vi "Teleop.vi"(10 "Match Info":T1={"Autonomous Elapsed Seconds"=0.0, "TeleOp Elapsed Seconds"=0.0, "Disabled Elapsed Seconds"=0.0, "Visited Autonomous"=FALSE, "Visited TeleOp"=FALSE, "Visited Disabled"=FALSE, "Autonomous Settings"={"Autonomous Style"=enum."Independent", "VI Refnum"=refnum}}, 11 "Call Context":T2) -> ()   [LabVIEW 2016]
doc: "This VI is called for each TeleOp packet received from the DS where the robot is not disabled. It is often used to read from the joysticks and update I/O or to update setpoints for timed control loops. It should complete and return within 20 milliseconds or it may miss DS packets."
uses:
  <vilib>/Rock Robotics/WPI/DriverStation/WPI_DriverStationDerivedRobotMode.ctl
  <vilib>/Rock Robotics/WPI/DriverStation/WPI_DriverStationMatch Info.ctl
  <vilib>/Rock Robotics/WPI/ThirdParty/CanMotor/TalonSRX/WPI_CANTalonSRX_APIFeedbackSelect.ctl
  <vilib>/Rock Robotics/WPI/ThirdParty/CanMotor/TalonSRX/WPI_CANTalonSRX_APIControlMode.ctl
  <vilib>/Rock Robotics/WPI/Utilities/WPI_GetSetVariantRefNum.vi
panel:
  out "SensorPosRotations":dbl
  out "Motor output Plot":cluster{"Applied Throttle":dbl}(graph)
  out "Target RPM":dbl
  out "SensorRPM Velocity RPM":dbl
  in  "Ramp Rate":dbl
  in  "I Zone":dbl
  in  "F":dbl
  in  "D":dbl
  in  "I":dbl
  in  "P":dbl
  out "Applied Output":dbl
  out "Speed Closed Loop Plots":cluster{dbl, "Sensor Velocity":dbl}(graph)
  # "Use the Left Y-axis on Logitech Gamepad.\n\nVelocityNativeUnits = Change In Sensor / 100mS\nalso\nVelocityNativeUnits = RPM / 600 * SensorUnitsPerRotation\n\nFgain = 100% X 1023 / VelocityNativeUnits , \n       where VelocityNativeUnits  is measured at 100% throttle\n\nMag Encoder has 4096 units per rotation.\n\nExample: VelocityRPM is 10198 at 100% throttle\n                 => VelocityNativeUnits = (10198 / 600 * 4096) = 69618\n                 => Fgain = (1023 / 69618)  = 0.01469"
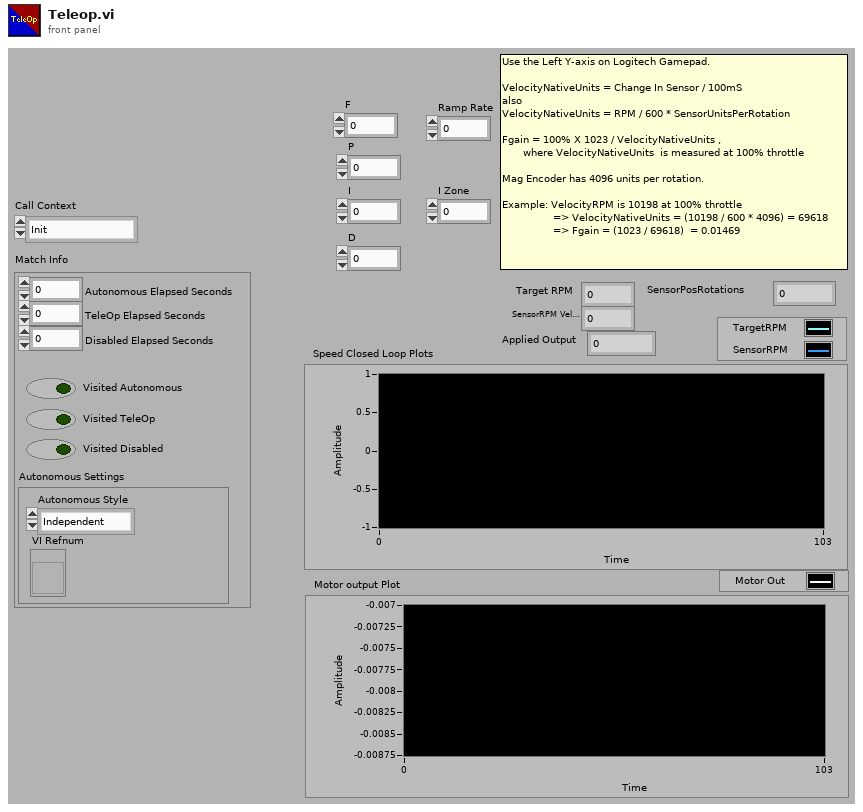
[diagram p1: front panel]
types:
  T1 = typedef "WPI_DriverStationMatch Info.ctl" = cluster{"Autonomous Elapsed Seconds":dbl, "TeleOp Elapsed Seconds":dbl, "Disabled Elapsed Seconds":dbl, "Visited Autonomous":bool, "Visited TeleOp":bool, "Visited Disabled":bool, "Autonomous Settings":cluster{"Autonomous Style":enum16{"Iterative", "Independent"}, "VI Refnum":refnum<vi>}}
  T2 = typedef "WPI_DriverStationDerivedRobotMode.ctl" = enum16{"Init", "Execute", "Stop"}
  T3 = typedef "WPI_CANTalonSRX_APIFeedbackSelect.ctl" = enum16{"Digital Quadrature Encoder", "Analog Potentiometer", "Analog Encoder", "Count on Quad-A (Rising-Edge)", "Count on Quad-A (Falling-Edge)", "CTR Magnetic Enc (Absolute)", "CTR Magnetic Enc (Relative)", "Pulse Width"}
  T4 = typedef "WPI_MotorControlDeviceRef.ctl" = cluster{"DeviceStatus":errorcluster, "Type":T5, "PWM":cluster{"PWM Channel":T6, "DeadBand":T7}, "CAN":cluster{"Device Number":u8, "SetOutput VI Ref":variant, "GetOutput VI Ref":variant, "Enable VI Ref":variant, "Disable VI Ref":variant, "Data":variant}, "Invert":bool}
  T5 = typedef "WPI_MotorControlType.ctl" = enum16{"PWM", "CAN"}
  T6 = typedef "FPGA_DIOPWMChannel.ctl" = enum8{"PWM 0", "PWM 1", "PWM 2", "PWM 3", "PWM 4", "PWM 5", "PWM 6", "PWM 7", "PWM 8", "PWM 9", "PWM MXP 0", "PWM MXP 1", "PWM MXP 2", "PWM MXP 3", "PWM MXP 4", "PWM MXP 5", "PWM MXP 6", "PWM MXP 7", "PWM MXP 8", "PWM MXP 9", "Invalid"}
  T7 = typedef "WPI_PWMDeadband.ctl" = cluster{"Name":string, "maxPositivePwm":i32, "minPositivePwm":i32, "centerPwm":i32, "maxNegativePwm":i32, "minNegativePwm":i32, "angularRange":u16}
  T8 = typedef "WPI_JoystickDevRef.ctl" = cluster{"Device":T9}
  T9 = typedef "WPI_JoystickDeviceEnum.ctl" = enum16{"USB 0", "USB 1", "USB 2", "USB 3", "USB 4", "USB 5"}
  T10 = typedef "WPI_CANTalonSRX_APIControlMode.ctl" = enum8{"Percent VBus", "Speed", "Position", "Slave", "Unchanged / Invalid", "Voltage Compensation", "Current", "Motion Profile", "Motion Magic"}
  T11 = typedef "WPI_CANTalonSRX_GlobalStatus.ctl" = cluster{"Applied Throttle":dbl, "Module Enabled":bool, "CAN Error":errorcluster, "Closed Loop Error":dbl, "Forward Limit Switch Closed":bool, "Reverse Limit Switch Closed":bool, "Sensor Position":dbl, "Sensor Velocity":dbl, "Current":dbl, "Sticky Fault - Over Temp":bool, "Sticky Fault - Under Voltage":bool, "Sticky Fault - Forward Limit":bool, "Sticky Fault - Reverse Limit":bool, "Sticky Fault - Forward Soft Limit":bool, "Sticky Fault - Reverse Soft Limit":bool, "Brake is Enabled":bool, "Encoder Position":dbl, "Encoder Velocity":dbl, "Encoder Index Count":dbl, "Encoder A Pin State":bool, "Encoder B Pin State":bool, "Encoder Index Pin State":bool, "Analog In":dbl, "Analog In Velocity":dbl, "Temperature (C)":dbl, "Battery Voltage":dbl, "Control 5 Is Supported":bool, "Current Profile Slot Select":dbl, "Pos Div 8":bool, "Vel Div 4":bool, "Pulse Width Position":i32, "Pulse Width Velocity":i32, "Pulse Width Rise To Rise (us)":i32, "Pulse Width Rise To Fall (us)":i32, "Mot Prof Active Is Under Run":bool, "Mot Prof Active Has Under Run":bool, "Mot Prof Active Is Last":bool, "Mot Prof Active Velocity Only":bool, "Mot Prof Active Is Valid":bool, "Mot Prof Buffer Is Full":bool, "Mot Prof Active Profile Slot Select":i32, "Mot Prof NextID":i32, "Mot Prof Count":i32, "Mot Prof Active Velocity":dbl, "Mot Prof Active Position":dbl, "Mot Prof Output Enable":i32, "UsageFrame":u32}
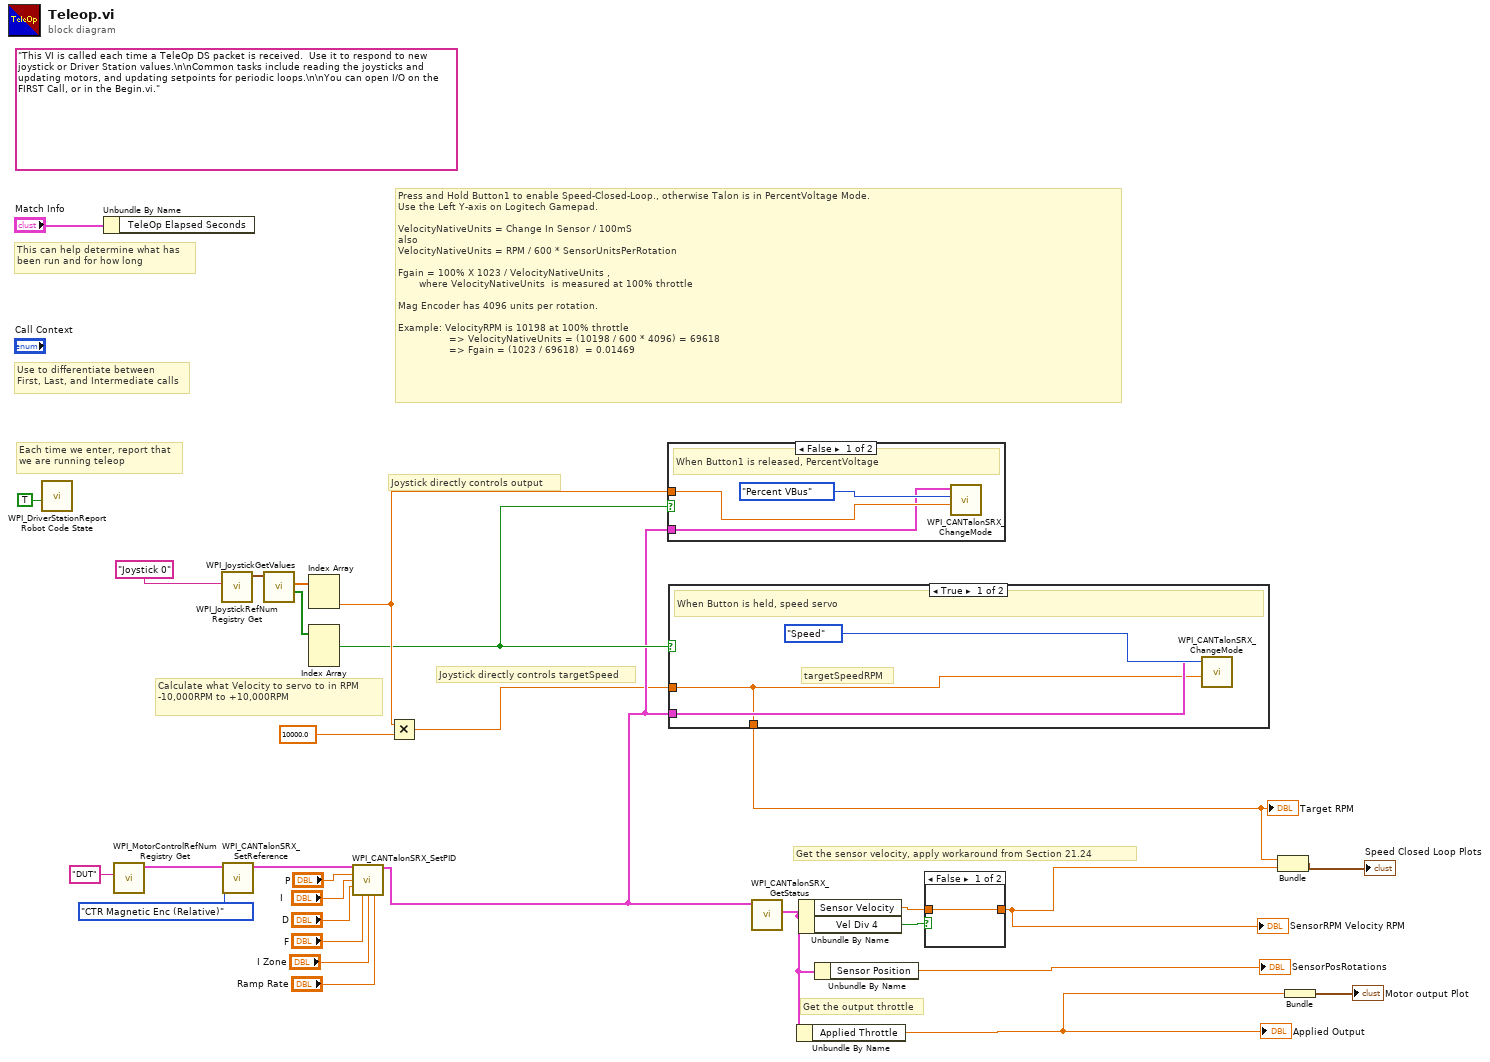
[diagram p0: block diagram]
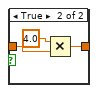
[diagram p2: hidden frame]
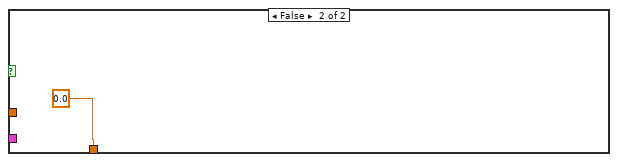
[diagram p4: hidden frame]
diagram:
  (unwired) "This VI is called each time a TeleOp DS packet is received.  Use it to respond to new joystick or Driver Station values.\n\nCommon tasks include reading the joysticks and updating motors, and updating setpoints for periodic loops.\n\nYou can open I/O on the FIRST Call, or in the Begin.vi."
  # "Press and Hold Button1 to enable Speed-Closed-Loop., otherwise Talon is in PercentVoltage Mode.  \nUse the Left Y-axis on Logitech Gamepad.\n\nVelocityNativeUnits = Change In Sensor / 100mS\nalso\nVelocityNativeUnits = RPM / 600 * SensorUnitsPerRotation\n\nFgain = 100% X 1023 / VelocityNativeUnits , \n       where VelocityNativeUnits  is measured at 100% throttle\n\nMag Encoder has 4096 units per rotation.\n\nExample: VelocityRPM is 10198 at 100% throttle\n                 => VelocityNativeUnits = (10198 / 600 * 4096) = 69618\n                 => Fgain = (1023 / 69618)  = 0.01469"
  # "Get the output throttle"
  # "Get the sensor velocity, apply workaround from Section 21.24"
  # "Joystick directly controls targetSpeed"
  # "Joystick directly controls output"
  # "Calculate what Velocity to servo to in RPM\n-10,000RPM to +10,000RPM"
  # "Each time we enter, report that\nwe are running teleop"
  # "Use to differentiate between\nFirst, Last, and Intermediate calls"
  # "This can help determine what has\nbeen run and for how long"
  n1 = call <vilib>:"WPI_DriverStationReport Robot Code State.vi"("TeleOp"=TRUE ("Autonomous")) -> ()  [unwired: 10 in, 1 out]
  n2 = Unbundle By Name("Match Info") -> ()  [unwired: 1 out]
  n3 = call <vilib>:"WPI_MotorControlRefNum Registry Get.vi"("refnum name"="DUT") -> ("MotorControlDevRef"=w10:T4)  [unwired: 9 in, 1 out]
  n4 = call <vilib>:"WPI_JoystickRefNum Registry Get.vi"("refnum name"="Joystick 0") -> ("JoystickDevRef"=w28:T8)  [unwired: 1 in, 9 out]
  n5 = call <vilib>:"WPI_CANTalonSRX_SetReference.vi"("Feedback Reference"=WPI_CANTalonSRX_APIFeedbackSelect."CTR Magnetic Enc (Relative)", "CAN Talon SRX Ref"=w10) -> ("CAN Talon SRX Ref"=w9:T4)  [unwired: 8 in, 1 out]
  n6 = call <vilib>:"WPI_JoystickGetValues.vi"("JoystickDevRef"=w28) -> ("Buttons"=w25:bool[], "Axes"=w26:dbl[])  [unwired: 6 in, 3 out]
  n7 = Index Array(array=w26) -> (element #2=w17:dbl)  [unwired: 2 in, 1 out]
  n8 = Index Array(array=w25) -> (element #1=w11:bool)  [unwired: 3 in, 2 out]
  n9 = call <vilib>:"WPI_CANTalonSRX_SetPID.vi"("CAN Talon SRX Ref"=w9, "P"="P", "I"="I", "D"="D", "F"="F", "I Zone"="I Zone", "Ramp Rate"="Ramp Rate") -> ("CAN Talon SRX Ref"=w5:T4)  [unwired: 7 in, 1 out]
  n10 = Multiply(x=w17, y=10000.0) -> (x*y=w2:dbl)
  n11 = case shown="False" w11 {
    tunnel: w17 -> [w32 _]
    tunnel: w5 -> [w31 _]
    frame False {
      # "When Button1 is released, PercentVoltage"
      n12 = call <vilib>:"WPI_CANTalonSRX_ChangeMode.vi"("Output"=w32, "Control Mode"=WPI_CANTalonSRX_APIControlMode."Percent VBus", "CAN Talon SRX Ref"=w31) -> ()  [unwired: 7 in, 2 out]
    }
    frame True {
    }
  }
  n13 = case shown="True" w11 {
    tunnel: w2 -> [w34 _]
    tunnel: w5 -> [w35 _]
    tunnel: [w34 0.0 ("x")] -> w1
    frame True {
      # "targetSpeedRPM"
      # "When Button is held, speed servo"
      n14 = call <vilib>:"WPI_CANTalonSRX_ChangeMode.vi"("Output"=w34, "Control Mode"=WPI_CANTalonSRX_APIControlMode."Speed", "CAN Talon SRX Ref"=w35) -> ()  [unwired: 7 in, 2 out]
    }
    frame False {
    }
  }
  "Target RPM" <- w1
  n15 = call <vilib>:"WPI_CANTalonSRX_GetStatus.vi"("CAN Talon SRX Ref"=w5) -> ("Talon SRX Status"=w7:T11)  [unwired: 8 in, 2 out]
  n16 = Unbundle By Name(w7) -> ("Applied Throttle"=w3:dbl)
  "Applied Output" <- w3
  n17 = Unbundle By Name(w7) -> ("Sensor Velocity"=w14:dbl, "Vel Div 4"=w13:bool)
  n18 = Unbundle By Name(w7) -> ("Sensor Position"=→"SensorPosRotations":dbl)
  n19 = case shown="False" w13 {
    tunnel: [w38 w40] -> w12
    tunnel: w14 -> [w38 w39]
    frame False {
    }
    frame True {
      n20 = Multiply(x=4.0, y=w39) -> (x*y=w40:dbl)
    }
  }
  "SensorRPM Velocity RPM" <- w12
  n21 = Bundle("x"=w1, "Sensor Velocity"=w12) -> (→"Speed Closed Loop Plots":cluster{"x":dbl, "Sensor Velocity":dbl})  [unwired: 1 in]
  n22 = Bundle("Applied Throttle"=w3) -> (→"Motor output Plot":cluster{"Applied Throttle":dbl})  [unwired: 1 in]
